vi "encode double.vi"(10 "double":dbl, 11 "byte array in":u8[](array[numeric]) format="%.0b") -> (3 "byte array out":u8[](array[numeric]))   [LabVIEW 2013, in "protocol buffers encoder.lvlib"]
uses:
  protocol buffers encoder.lvlib
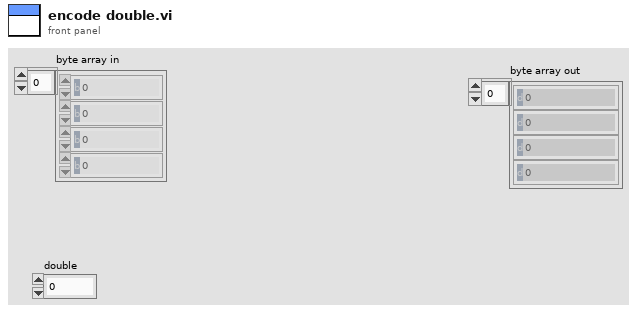
[diagram p1: front panel]
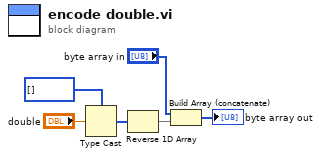
[diagram p0: block diagram]
diagram:
  n1 = Type Cast(type=u8[] [] ("byte array in"), x="double") -> (*(type *) &x=w5:u8[])
  n2 = Reverse 1D Array(array=w5) -> (reversed array=w2:u8[])
  n3 = Build Array (concatenate)("byte array in", w2) -> (→"byte array out":u8[])
